vi "Lockin.vi"(4 "stop?":bool, 6 "initialize?":bool, 8 "error in (no error)":errorcluster, 11 "Transport":refnum<class "SMO.Transport.lvclass">) -> (0 "error out":errorcluster, 3 "Transport out":refnum<class "SMO.Transport.lvclass">)   [LabVIEW 2019, in "SMO.Transport.lvclass"]
uses:
  SMO.Transport.lvclass
  <userlib>/LevyLab/Instrument Framework/Instrument Types/Cryostat/Instrument.Cryostat.lvclass
  Control Experiment/Control Experiment.lvclass
  <userlib>/LevyLab/Krohn Hite 7008/Instrument.KH7008.lvclass
  <userlib>/LevyLab/Lockin-Multichannel/Instrument.Lockin/Instrument.Lockin.lvclass
  Control Experiment/Typedefs/Instruments--cluster.ctl
  <userlib>/LevyLab/Instrument Framework/Instrument Types/VSource/Instrument.VSource.lvclass
  <userlib>/LevyLab/Instrument Framework/Instrument Types/VNA/Instrument.VNA.lvclass
  <userlib>/LevyLab/Instrument Framework/Instrument Types/Strain/Instrument.Strain.lvclass
  <userlib>/LevyLab/Instrument Framework/Instrument Types/CBridge/Instrument.CBridge.lvclass
  SMO.SweepControl/SMO.SweepControl.lvclass
  SMO.Control Experiment/SMO.Control Experiment.lvclass
  C:/Program Files (x86)/National Instruments/LabVIEW 2019/user.lib/LevyLab/Instrument Framework/SMOs/Instrument/Instrument.lvclass
  C:/Program Files (x86)/National Instruments/LabVIEW 2019/vi.lib/JKI/JKI SMO/SMO/SMO.lvclass
  <userlib>/LevyLab/Instrument Framework/Instrument Types/Delay Line/Instrument.DelayLine.lvclass
panel:
  in  "Tab Control":enum32{"lockin/SG Control", "Data", "Other"}(tab)
  out "elapsed time (s)":u32=76
  in  "Experiment Comments":string="describe only the experiment you're doing right now"
  in  "Experiment Folder":string="Experiment folder"
  out "T (mK)":dbl
  out "Field (T)":dbl=0.5 format="%#_13g"
  out "time b/w points (ms)":u32=76
  in  "stop":bool
  out "x-y":u32
  out "X Lockins":cluster{dbl[], dbl[]}[](graph)
  out "Y Lockins":cluster{dbl[], dbl[]}[](graph)
  out "G4T":cluster{dbl[], dbl[]}[](graph)
  # "*** These controls are only read if this VI is the top level. If is is called from Sweep Control then the folder and comments come from Sweep Control.vi ***"
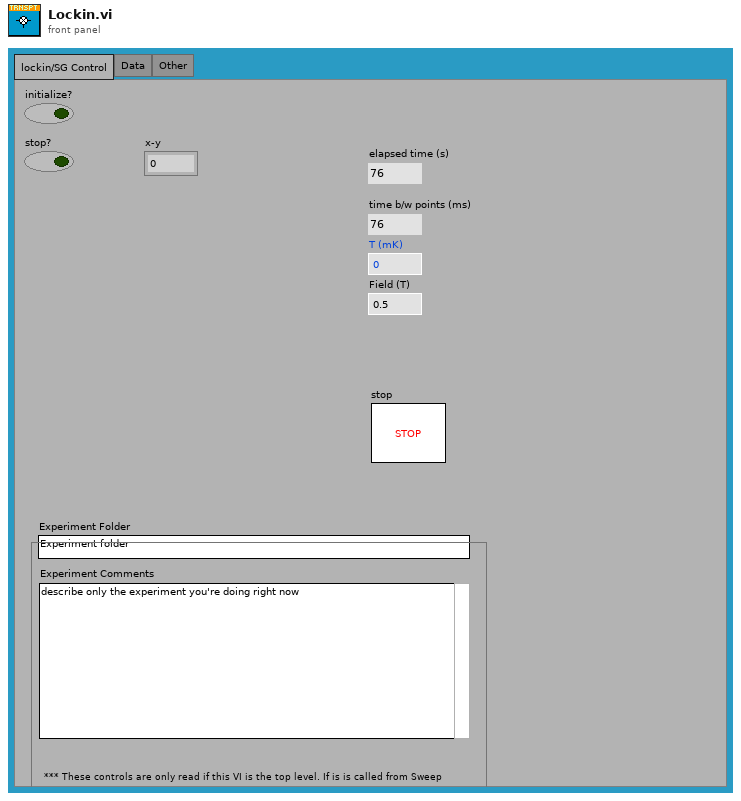
[diagram p1: front panel]
types:
  T1 = enum32{"Invalid", "Standard", "Closed", "Hidden", "Minimized", "Maximized"}
  T2 = enum32{"invalid app kind", "Development System", "Run Time System", "Student Edition", "Embedded LabVIEW", "Evaluation", "Custom"}
  T3 = typedef "Control Experiment.lvclass/Instruments--cluster.ctl" = cluster{"KH7008":refnum<class "Instrument.KH7008.lvclass">[], "Lockin":refnum<class "Instrument.Lockin.lvclass">, "Temperature":refnum<class "Instrument.Cryostat.lvclass">, "Magnet":refnum<class "Instrument.Cryostat.lvclass">, "Rotator":refnum<class "Instrument.Cryostat.lvclass">, "Level":refnum<class "Instrument.Cryostat.lvclass">, "Capacitance Bridge":refnum<class "Instrument.CBridge.lvclass">, "Delay Line":refnum<class "Instrument.DelayLine.lvclass">, "Strain Cell":refnum<class "Instrument.Strain.lvclass">, "VNA":refnum<class "Instrument.VNA.lvclass">, "Voltage Source":refnum<class "Instrument.VSource.lvclass">}
  T4 = cluster{"Core":cluster{"Current VI Reference":refnum<vi>, "Close Panel on Exit?":bool}, "Transport":refnum<class "SMO.Transport.lvclass">, "Control Experiment":refnum<class "SMO.Control Experiment.lvclass">, "Instruments":T3, "Results (Dictionary)":cluster{"key":string, "value":dbl}[], "ms [0]":u32, "ms [i]":u32, "Execution:State":enum32{"Bad", "Idle", "Run top level", "Running"}}
  T5 = enum32{"Bad", "Idle", "Run top level", "Running"}
  T6 = cluster{"Current VI Reference":refnum<vi>, "Close Panel on Exit?":bool}
  T7 = cluster{"I-":i32, "I+":i32, "V1-":i32, "V1+":i32, "I2-":i32, "I2+":i32, "V2-":i32, "V2+":i32}
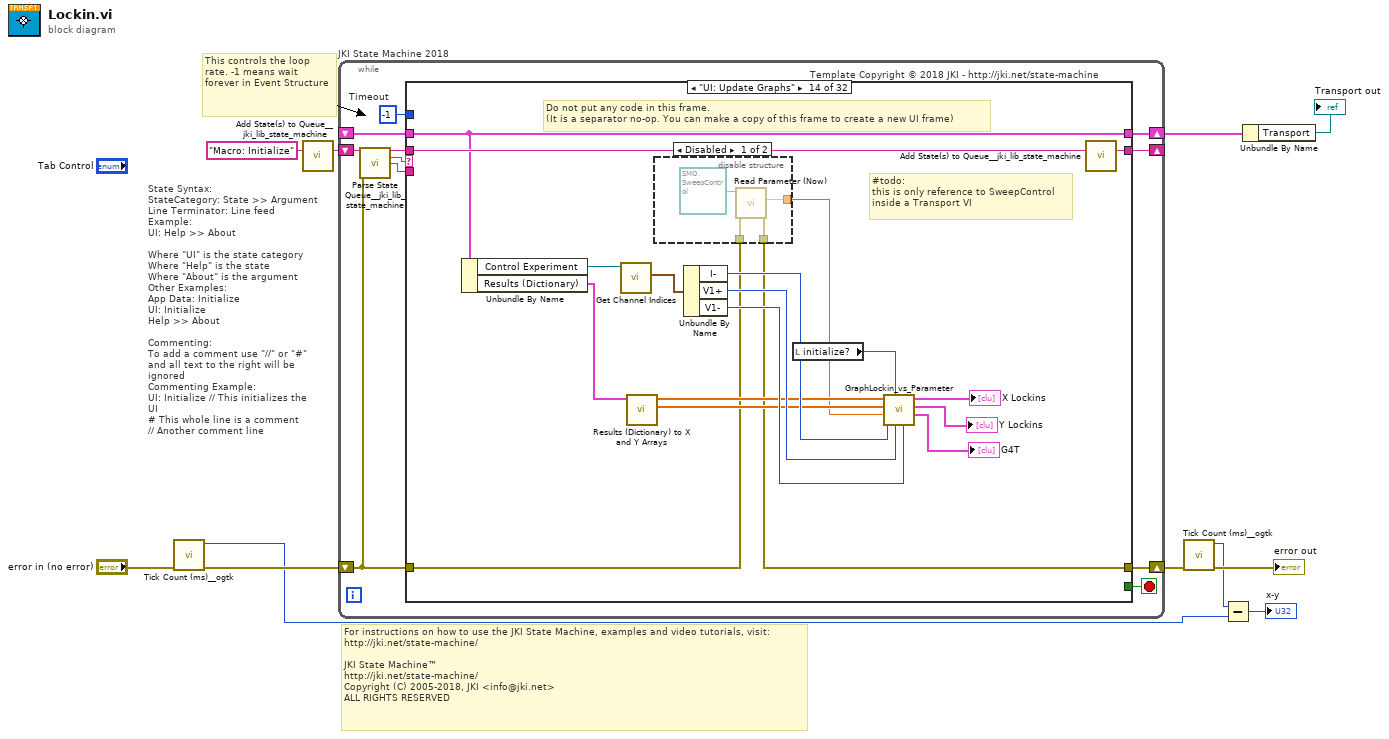
[diagram p0: block diagram]
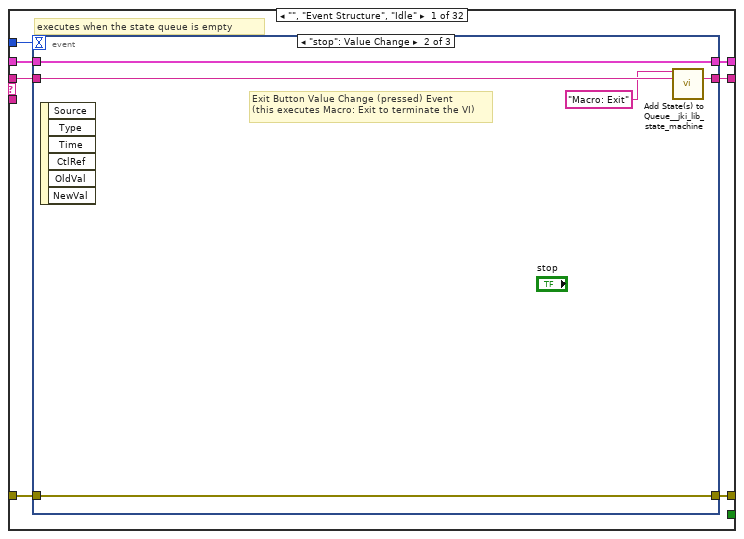
[diagram p2: hidden frame]
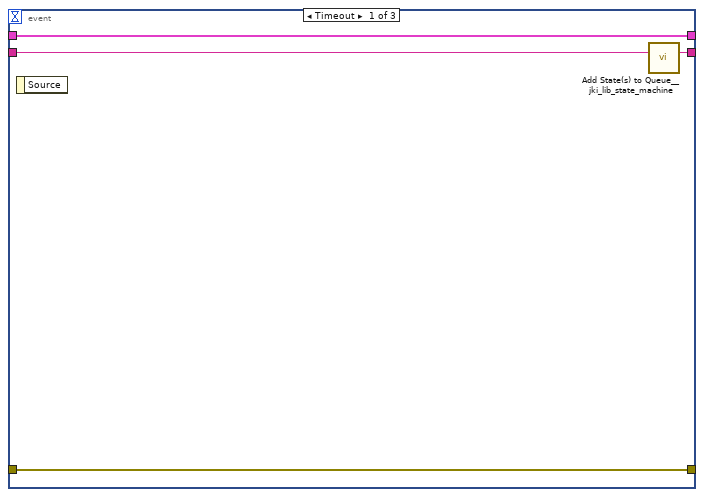
[diagram p3: hidden frame]
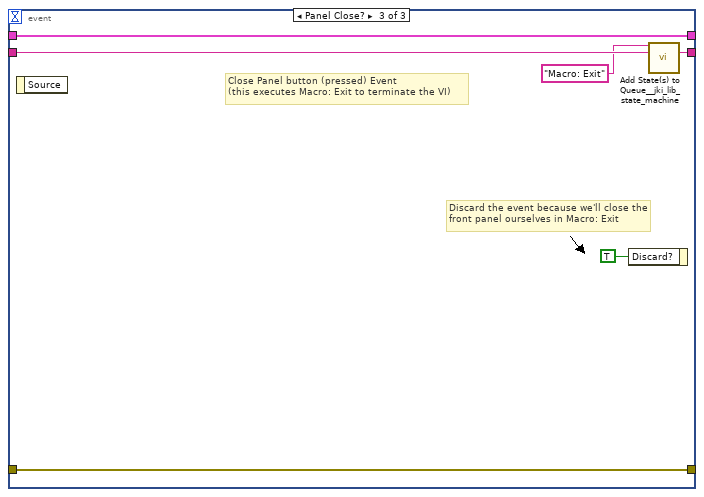
[diagram p4: hidden frame]
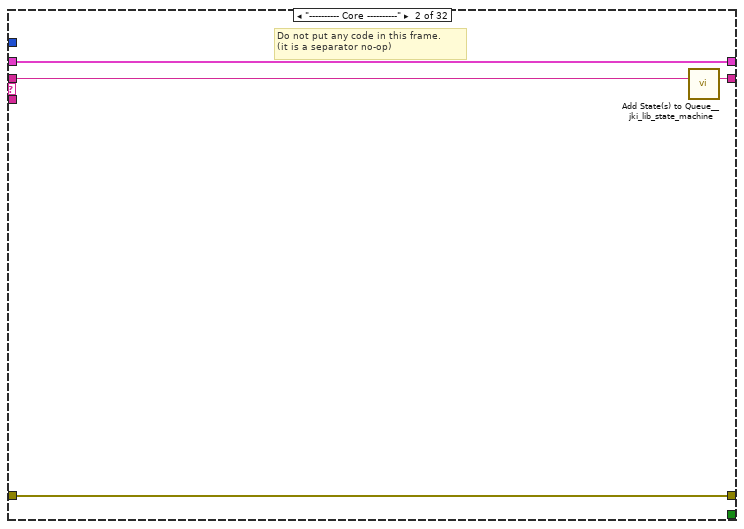
[diagram p5: hidden frame]
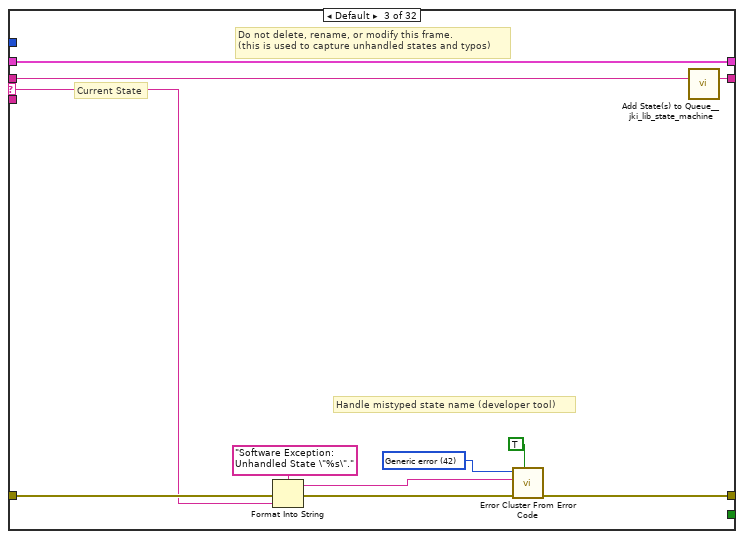
[diagram p6: hidden frame]
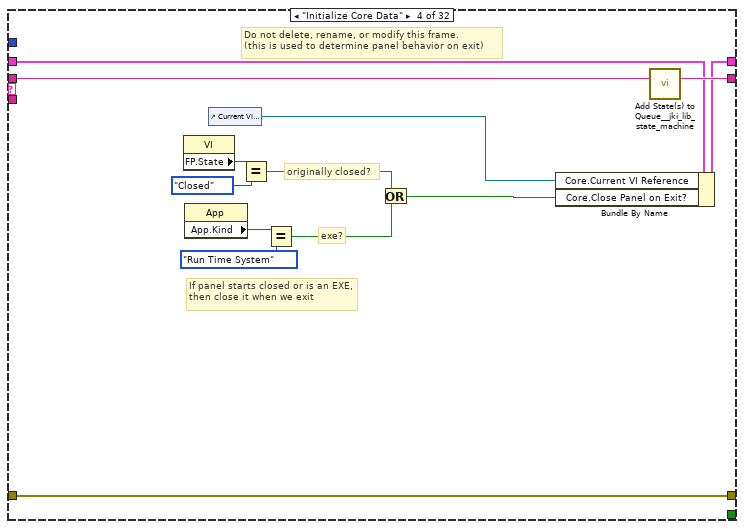
[diagram p7: hidden frame]
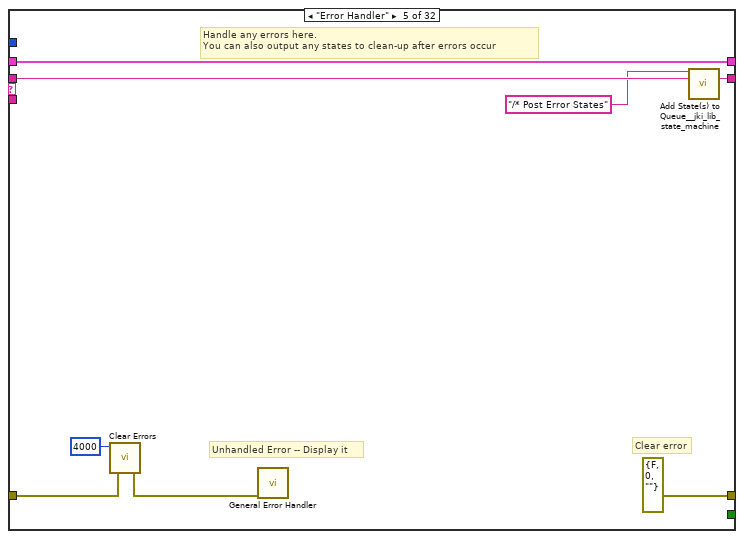
[diagram p8: hidden frame]
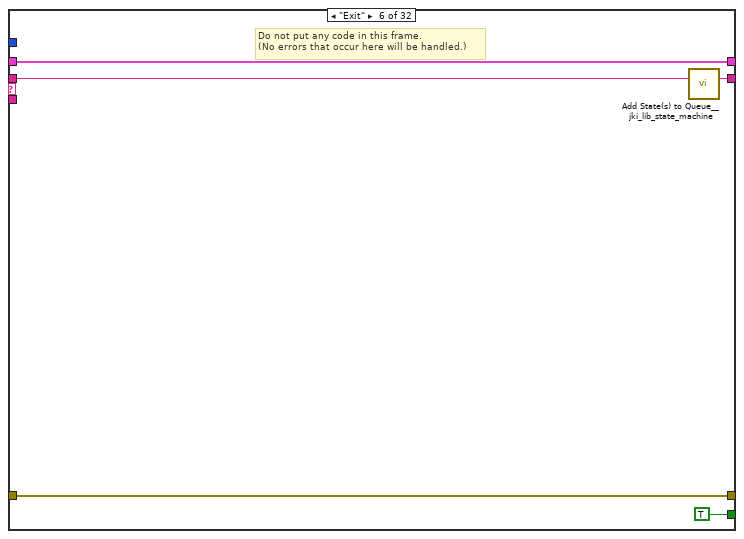
[diagram p9: hidden frame]
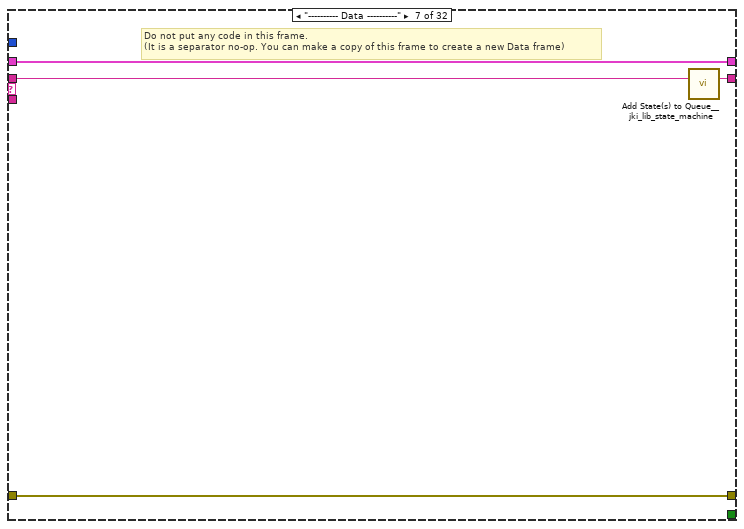
[diagram p10: hidden frame]
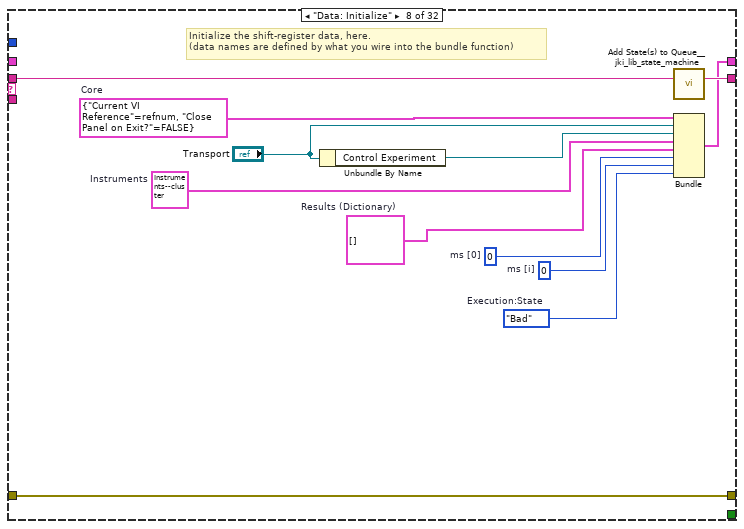
[diagram p11: hidden frame]
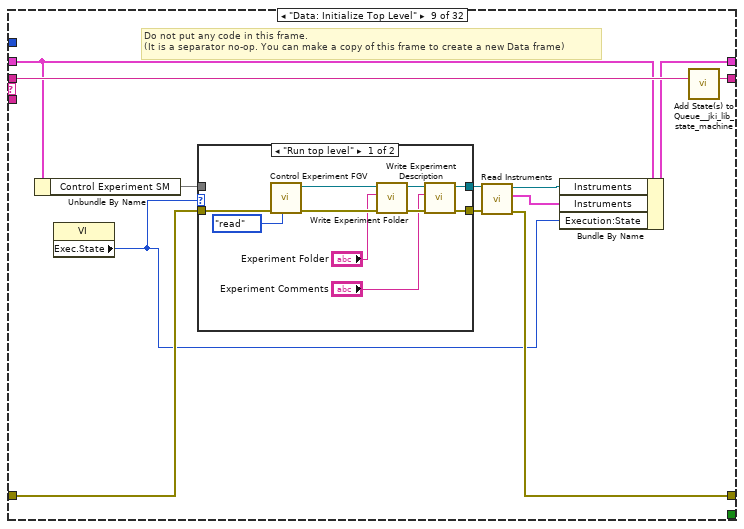
[diagram p12: hidden frame]
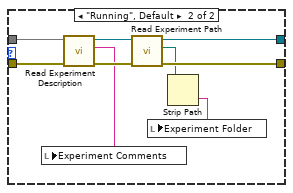
[diagram p13: hidden frame]
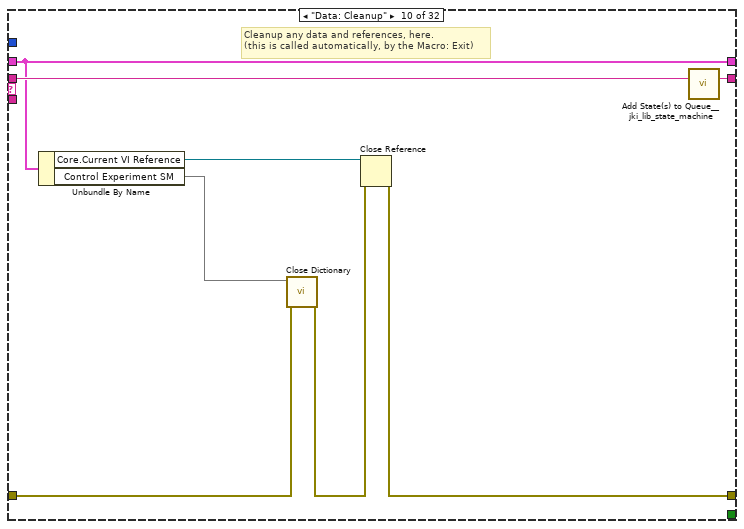
[diagram p14: hidden frame]
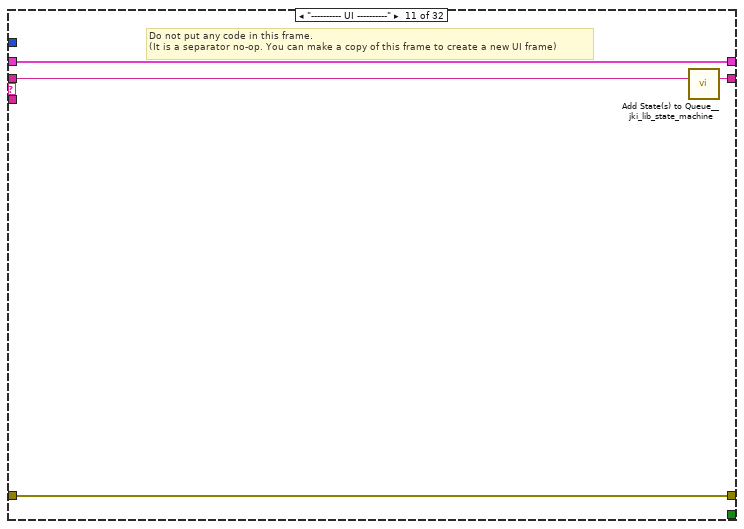
[diagram p15: hidden frame]
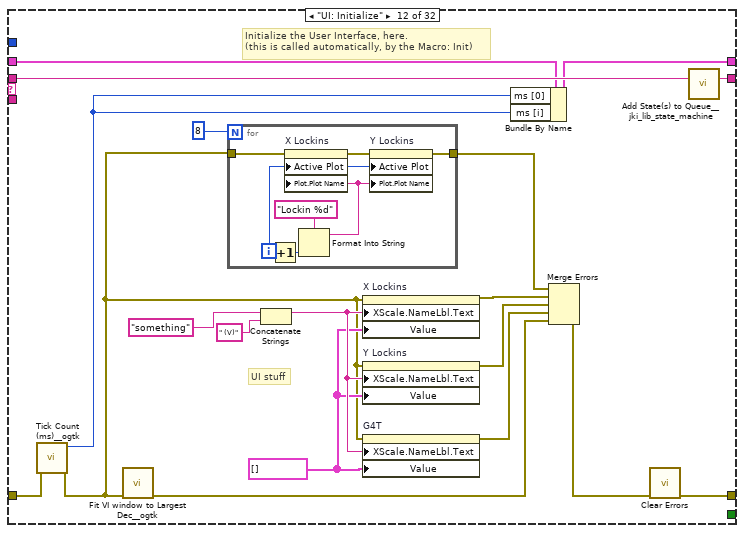
[diagram p16: hidden frame]
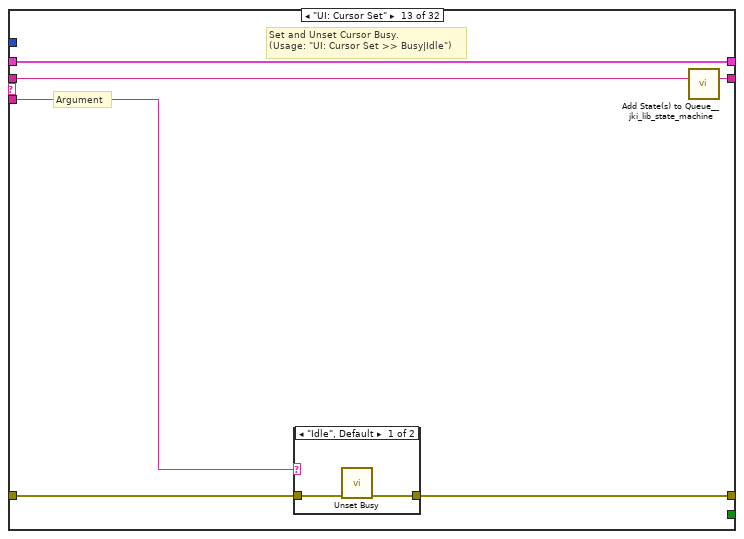
[diagram p17: hidden frame]
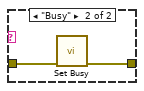
[diagram p18: hidden frame]
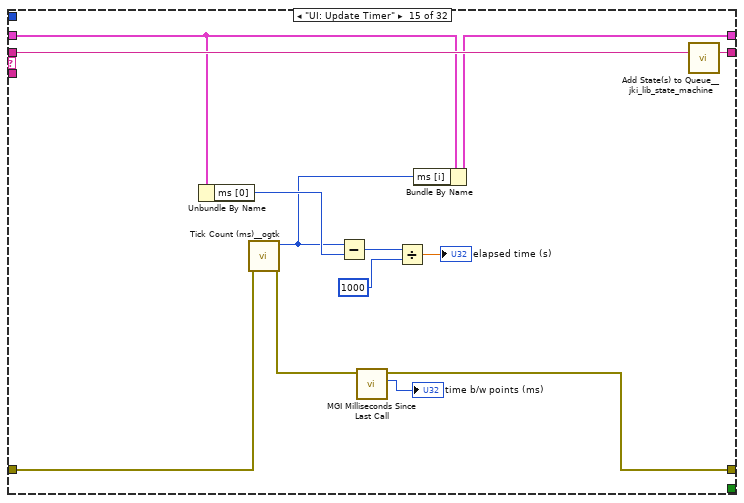
[diagram p20: hidden frame]
diagram:
  # "For instructions on how to use the JKI State Machine, examples and video tutorials, visit:\nhttp://jki.net/state-machine/\n\nJKI State Machine™\nhttp://jki.net/state-machine/\nCopyright (C) 2005-2018, JKI <info@jki.net>\nALL RIGHTS RESERVED"
  # "State Syntax:\nStateCategory: State >> Argument\nLine Terminator: Line feed\nExample:\nUI: Help >> About\n\nWhere \"UI\" is the state category\nWhere \"Help\" is the state\nWhere \"About\" is the argument\nOther Examples:\nApp Data: Initialize\nUI: Initialize\nHelp >> About\n\nCommenting:\nTo add a comment use \"//\" or \"#\" and all text to the right will be ignored\nCommenting Example:\nUI: Initialize // This initializes the UI\n# This whole line is a comment\n// Another comment line"
  # "This controls the loop rate. -1 means wait forever in Event Structure"
  n1 = call <userlib>:"Tick Count (ms)__ogtk.vi"("error in (no error)"="error in (no error)") -> ("error out"=w6:errorcluster, "millisecond timer value"=w2:u32)  [unwired: 9 in]
  n2 = call <vilib>:"Add State(s) to Queue__jki_lib_state_machine.vi"("State(s) in (\"\")"="Macro: Initialize") -> ("States Out"=w11:string)  [unwired: 14 in]
  n3 = while "JKI State Machine 2018" {
    shift-right: [w15] -> w9
    shift-left: _ -> [w14]
    shift-right: [w18] -> w5
    shift-left: w6 -> [w12]
    shift-right: [w17] -> _
    shift-left: w11 -> [w19]
    stop <- w16 stop-if-true
    w13 = -1  # Timeout
    # "Template Copyright © 2018 JKI - http://jki.net/state-machine"
    n4 = call <vilib>:"Parse State Queue__jki_lib_state_machine.vi"("State Queue"=w19, "Error In (no error)"=w12) -> ("Remaining States"=w21:string, "Current State"=w22:string, "Arguments"=w20:string)  [unwired: 11 in]
    n5 = case shown="\"UI: Update Graphs\"" w22 {
      selector: w22 -> [_ _ w49 _ _ _ _ _ _ _ _ _ _ _ _ _ _ _ _ _ _ _ _ _ _ _ _ _ _ _ _ _]
      tunnel: w21 -> [w29 w48 w53 w72 w80 w85 w89 w101 w113 w140 w144 w163 w176 w198 w216 w223 w292 w300 w314 w324 w328 w332 w338 w342 w354 w366 w378 w391 w418 w422 w426 w434]
      tunnel: w20 -> [_ _ _ _ _ _ _ _ _ _ _ _ w171 _ _ w217 _ _ _ _ _ _ _ _ _ _ _ _ _ _ _ _]
      tunnel: w14 -> [w27 w45 w51 w65 w77 w83 w86 _ w104 w136 w141 w150 w174 w186 w211 w219 w289 w298 w311 w321 w325 w329 w336 w339 w350 w363 w367 w386 w414 w419 w423 w432]
      tunnel: [w26 w46 w55 w69 errorcluster {"status"=FALSE, "code"=0, "source"=""} ("error out") w82 w87 w98 w105 w137 w142 w154 w172 w183 w205 w220 w290 w297 w312 w322 w326 w330 w334 w340 w346 w355 w369 w381 w409 w420 w424 w429] -> w18
      tunnel: w12 -> [w25 w46 w54 w69 w74 w82 w87 w98 w106 w134 w142 w151 w173 w184 w213 w221 w290 w297 w312 w322 w326 w330 w335 w340 w351 w360 w370 w389 w410 w420 w424 w430]
      tunnel: [w28 w47 w52 w71 w79 w84 w88 w100 w112 w139 w143 w162 w175 w197 w215 w222 w291 w299 w313 w323 w327 w331 w337 w341 w353 w365 w377 w390 w417 w421 w425 w433] -> w17
      tunnel: [_ _ _ _ _ TRUE _ _ _ _ _ _ _ _ _ _ _ _ _ _ _ _ _ _ _ _ _ _ _ _ _ _] -> w16
      tunnel: [w24 w45 w51 w70 w77 w83 w86 w99 w103 w136 w141 w149 w174 w186 w210 w219 w289 w298 w311 w321 w325 w329 w336 w339 w349 w362 w372 w387 w415 w419 w423 w432] -> w15
      tunnel: w13 -> [w23 _ _ _ _ _ _ _ _ _ _ _ _ _ _ _ _ _ _ _ _ _ _ _ _ _ _ _ _ _ _ _]
      frame "", "Event Structure", "Idle" {
        # "executes when the state queue is empty"
        n6 = event shown="[1] \"stop\": Value Change" {
          selector: _ -> [_ _ _]
          dyn-events: _ -> [_ _ _]
          timeout: w23 -> [_ _ _]
          tunnel: w29 -> [w33 w38 w44]
          tunnel: [w32 w37 w43] -> w28
          tunnel: w27 -> [w30 w35 w41]
          tunnel: [w31 w36 w42] -> w26
          tunnel: w25 -> [w31 w36 w42]
          tunnel: [w30 w35 w41] -> w24
          event Timeout {
            n7 = event-data() -> ()  [unwired: 1 in, 1 out]
            n8 = call <vilib>:"Add State(s) to Queue__jki_lib_state_machine.vi"("State(s) in (\"\")"=w33) -> ("States Out"=w32:string)  [unwired: 14 in]
          }
          event "stop": Value Change {
            # "Exit Button Value Change (pressed) Event\n(this executes Macro: Exit to terminate the VI)"
            n9 = event-data() -> ()  [unwired: 1 in, 6 out]
            n10 = call <vilib>:"Add State(s) to Queue__jki_lib_state_machine.vi"("State(s) in Front (\"\")"="Macro: Exit", "State(s) in (\"\")"=w38) -> ("States Out"=w37:string)  [unwired: 13 in]
          }
          event Panel Close? {
            # "Discard the event because we'll close the front panel ourselves in Macro: Exit"
            # "Close Panel button (pressed) Event\n(this executes Macro: Exit to terminate the VI)"
            n11 = event-data() -> ()  [unwired: 1 in, 1 out]
            n12 = event-data("Discard?"=TRUE) -> ()  [unwired: 1 in, 1 out]
            n13 = call <vilib>:"Add State(s) to Queue__jki_lib_state_machine.vi"("State(s) in Front (\"\")"="Macro: Exit", "State(s) in (\"\")"=w44) -> ("States Out"=w43:string)  [unwired: 13 in]
          }
        }
      }
      frame "---------- Core ----------" {
        # "Do not put any code in this frame.\n(it is a separator no-op)"
        n14 = call <vilib>:"Add State(s) to Queue__jki_lib_state_machine.vi"("State(s) in (\"\")"=w48) -> ("States Out"=w47:string)  [unwired: 14 in]
      }
      frame Default {
        w58 = 42 items=["No error", "Argument error", "Memory is full", "Out of zone", "End of file", "File already open", "Generic file I/O error", "File not found", "File permission error", "Disk is full", "Duplicate path", "Too many files open", "System feature not enabled", "Resource file not found", "Cannot add resource", "Resource not found", "Image not found", "Image memory error", "Pen does not exist", "Config type invalid", "Config token not found", "Config parse error", "Config memory error", "Bad external code format", "Bad external code offset", "External code not present", "Null window", "Destroy window error", "Null menu", "Print aborted", "Bad print record", "Print driver error", "Windows error during printing", "Memory error during printing", "Print dialog error", "Generic print error", "Invalid device refnum", "Device not found", "Device parameter error", "Device unit error", "Cannot open device", "Device call aborted", "Generic error", "Cancelled by user", "Object ID too low", "Object ID too high", "Object not in heap", "Unknown heap", "Unknown object (invalid DefProc)", "Unknown object (DefProc not in table)", "Message out of range", "Invalid (null) method", "Unknown message", "Manager call not supported", "Bad address", "Network operation in progress", "Network operation timed out", "Connection is busy", "Network attribute not supported", "Network error", "Address in use", "System out of memory", "Connection aborted", "Connection refused", "Not connected", "Already connected", "Connection closed", "Initialization error (interapplication manager)", "Bad occurrence", "Wait on unbound occurrence handler", "Occurrence queue overflow", "Datalog type conflict", "Unused", "Unrecognized type (interapplication manager)", "Memory corrupt", "Failed to make temporary DLL", "Old CIN version", "Drag socket not found", "Failed to load drop-object", "Failed to register OLE object", "Failed to release OLE object", "Format specifier type mismatch", "Unknown format specifier", "Too few format specifiers", "Too many format specifiers", "Scan failed", "Newer CIN version", "Error converting to variant", "Runtime menu error", "Password tampered", "Variant attribute not found", "Incompatible variant data type", "Event data is not available", "Event Store is not present", "Occurrence is not found", "Event Queue is not created", "Event info is not available", "Refnum passed is NULL", "Error retrieving Class GUID", "Error retrieving CoClass GUID", "Error retrieving TypeLib GUID.", "Bad built application magic bytes.", "Specific driver is different from the specific driver associated with the Logical Name.", "There is no session opened to the class driver.", "Max Error", "MAX - Error with config objects", "MAX - Error loading configuration", "MAX - Group not supported"]
        # "Current State"
        # "Do not delete, rename, or modify this frame.\n(this is used to capture unhandled states and typos)"
        # "Handle mistyped state name (developer tool)"
        n15 = Format Into String(format string="Software Exception: Unhandled State \"%s\"." ("message"), error in=w54, w49) -> (resulting string=w57:string, error out=w56:errorcluster)  [unwired: 1 in]
        n16 = call <vilib>:"Error Cluster From Error Code.vi"("show call chain? (False)"=TRUE, "error in (no error)"=w56, "error message (\"\")"=w57, "error code (0)"=w58) -> ("error out"=w55:errorcluster)  [unwired: 5 in]
        n17 = call <vilib>:"Add State(s) to Queue__jki_lib_state_machine.vi"("State(s) in (\"\")"=w53) -> ("States Out"=w52:string)  [unwired: 14 in]
      }
      frame "Initialize Core Data" {
        # "Do not delete, rename, or modify this frame.\n(this is used to determine panel behavior on exit)"
        # "originally closed?"
        # "exe?"
        # "If panel starts closed or is an EXE, then close it when we exit"
        n18 = property class="VI"() -> ("FP.State"=w62:T1)  [unwired: 2 in, 2 out]
        n19 = property class="App"() -> ("App.Kind"=w68:T2)  [unwired: 2 in, 2 out]
        n20 = control-ref of="Current VI Reference"() -> (w63:refnum<vi>)
        n21 = Equal?(x=w62, y=T1."Closed" ("Front Panel Window:State")) -> (x = y?=w60:bool)
        n22 = Equal?(x=w68, y=T2."Run Time System" ("Application:Kind")) -> (x = y?=w66:bool)
        n23 = Or(x=w60, y=w66) -> (x .or. y?=w64:bool)
        n24 = Bundle By Name(cluster=w65, "Core.Current VI Reference"=w63, "Core.Close Panel on Exit?"=w64) -> (w70:T4)
        n25 = call <vilib>:"Add State(s) to Queue__jki_lib_state_machine.vi"("State(s) in (\"\")"=w72) -> ("States Out"=w71:string)  [unwired: 14 in]
      }
      frame "Error Handler" {
        # "Unhandled Error -- Display it"
        # "Handle any errors here.\nYou can also output any states to clean-up after errors occur"
        # "Clear error"
        n26 = call <vilib>:"Clear Errors.vi"("error in (no error)"=w74, "specific error code to clear (0: all)"=4000) -> ("error out"=w73:errorcluster)  [unwired: 4 in, 1 out]
        n27 = call <vilib>:"General Error Handler.vi"("error in (no error)"=w73) -> ()  [unwired: 10 in, 5 out]
        n28 = call <vilib>:"Add State(s) to Queue__jki_lib_state_machine.vi"("State(s) in Front (\"\")"="/* Post Error States", "State(s) in (\"\")"=w80) -> ("States Out"=w79:string)  [unwired: 13 in]
      }
      frame "Exit" {
        # "Do not put any code in this frame.\n(No errors that occur here will be handled.)"
        n29 = call <vilib>:"Add State(s) to Queue__jki_lib_state_machine.vi"("State(s) in (\"\")"=w85) -> ("States Out"=w84:string)  [unwired: 14 in]
      }
      frame "---------- Data ----------" {
        # "Do not put any code in this frame.\n(It is a separator no-op. You can make a copy of this frame to create a new Data frame)"
        n30 = call <vilib>:"Add State(s) to Queue__jki_lib_state_machine.vi"("State(s) in (\"\")"=w89) -> ("States Out"=w88:string)  [unwired: 14 in]
      }
      frame "Data: Initialize" {
        w90 = cluster{"key":string, "value":dbl}[] []  # Results (Dictionary)
        w91 = T5."Bad"  # Execution:State
        w93 = u32 0  # ms [i]
        w94 = u32 0  # ms [0]
        w95 = T3 {"KH7008"=[], "Lockin"=refnum, "Temperature"=refnum, "Magnet"=refnum, "Rotator"=refnum, "Level"=refnum, "Capacitance Bridge"=refnum, "Delay Line"=refnum, "Strain Cell"=refnum, "VNA"=refnum, "Voltage Source"=refnum}  # Instruments
        w97 = T6 {"Current VI Reference"=refnum, "Close Panel on Exit?"=FALSE}  # Core
        # "Initialize the shift-register data, here.\n(data names are defined by what you wire into the bundle function)"
        n31 = Unbundle By Name("Transport") -> ("Control Experiment"=w92:refnum<class "SMO.Control Experiment.lvclass">)
        n32 = call <vilib>:"Add State(s) to Queue__jki_lib_state_machine.vi"("State(s) in (\"\")"=w101) -> ("States Out"=w100:string)  [unwired: 14 in]
        n33 = Bundle("Core"=w97, "Transport"="Transport", "Control Experiment"=w92, "Instruments"=w95, "Results (Dictionary)"=w90, "ms [0]"=w94, "ms [i]"=w93, "Execution:State"=w91) -> (w99:T4)  [unwired: 1 in]
      }
      frame "Data: Initialize Top Level" {
        # "Do not put any code in this frame.\n(It is a separator no-op. You can make a copy of this frame to create a new Data frame)"
        n34 = Unbundle By Name(w104) -> ("Control Experiment SM"=w107)
        n35 = property class="VI"() -> ("Exec.State"=w102:T5)  [unwired: 2 in, 2 out]
        n36 = case shown="\"Run top level\"" w102 {
          tunnel: w106 -> [w123 w131]
          tunnel: [w118 w127] -> w108
          tunnel: [w117 w128] -> w109
          tunnel: w107 -> [_ w132]
          frame "Run top level" {
            n37 = call "Control Experiment FGV.vi"("Function"=enum16{"read", "write"}."read", "error in (no error)"=w123) -> ("error out"=w121:errorcluster, "Control Experiment.lvclass out"=w122:refnum<class "Control Experiment.lvclass">)  [unwired: 8 in]
            n38 = call "Write Experiment Folder.vi"("error in (no error)"=w121, "Experiment Folder"="Experiment Folder", "Control Experiment in"=w122) -> ("error out"=w119:errorcluster, "Control Experiment out"=w120:refnum<class "Control Experiment.lvclass">)  [unwired: 7 in]
            n39 = call "Write Experiment Description.vi"("error in (no error)"=w119, "Experiment Description"="Experiment Comments", "Control Experiment in"=w120) -> ("error out"=w118:errorcluster, "Control Experiment out"=w117:refnum<class "Control Experiment.lvclass">)  [unwired: 7 in]
          }
          frame "Running", Default {
            n40 = call "Read Experiment Description.vi"("error in (no error)"=w131, "Control Experiment in"=w132) -> ("error out"=w130:errorcluster, "Experiment Description"=w125:string, "Control Experiment out"=w129:refnum<class "Control Experiment.lvclass">)  [unwired: 7 in]
            n41 = local write "Experiment Comments"(w125) -> ()
            n42 = call "Read Experiment Path.vi"("error in (no error)"=w130, "Control Experiment in"=w129) -> ("error out"=w127:errorcluster, "Experiment Path"=w126:path, "Control Experiment out"=w128:refnum<class "Control Experiment.lvclass">)  [unwired: 7 in]
            n43 = Strip Path(path=w126) -> (name=w124:string)  [unwired: 1 out]
            n44 = local write "Experiment Folder"(w124) -> ()
          }
        }
        n45 = call "Read Instruments.vi"("error in (no error)"=w108, "Control Experiment in"=w109) -> ("error out"=w105:errorcluster, "Instruments"=w111:T3, "Control Experiment out"=w110:refnum<class "Control Experiment.lvclass">)  [unwired: 7 in]
        n46 = Bundle By Name(cluster=w104, "Instruments"=w110, "Instruments"=w111, "Execution:State"=w102) -> (w103:T4)
        n47 = call <vilib>:"Add State(s) to Queue__jki_lib_state_machine.vi"("State(s) in (\"\")"=w113) -> ("States Out"=w112:string)  [unwired: 14 in]
      }
      frame "Data: Cleanup" {
        # "Cleanup any data and references, here.\n(this is called automatically, by the Macro: Exit)"
        n48 = Unbundle By Name(w136) -> ("Core.Current VI Reference"=w138:refnum<vi>, "Control Experiment SM"=w135)
        n49 = call "Close Dictionary.vi"("error in (no error)"=w134, "Control Experiment in"=w135) -> ("error out"=w133:errorcluster)  [unwired: 8 in, 1 out]
        n50 = Close Reference(reference=w138, error in (no error)=w133) -> (error out=w137:errorcluster)
        n51 = call <vilib>:"Add State(s) to Queue__jki_lib_state_machine.vi"("State(s) in (\"\")"=w140) -> ("States Out"=w139:string)  [unwired: 14 in]
      }
      frame "---------- UI ----------" {
        # "Do not put any code in this frame.\n(It is a separator no-op. You can make a copy of this frame to create a new UI frame)"
        n52 = call <vilib>:"Add State(s) to Queue__jki_lib_state_machine.vi"("State(s) in (\"\")"=w144) -> ("States Out"=w143:string)  [unwired: 14 in]
      }
      frame "UI: Initialize" {
        w147 = cluster{dbl[], dbl[]}[] [] ("G4T")
        # "UI stuff"
        # "Initialize the User Interface, here.\n(this is called automatically, by the Macro: Init)"
        n53 = call <userlib>:"Tick Count (ms)__ogtk.vi"("error in (no error)"=w151) -> ("error out"=w145:errorcluster, "millisecond timer value"=w148:u32)  [unwired: 9 in]
        n54 = call <userlib>:"Fit VI window to Largest Dec__ogtk.vi"("error in (no error)"=w145) -> ("error out"=w153:errorcluster)  [unwired: 5 in, 1 out]
        n55 = for {
          N: 8 -> [_]
          tunnel: [w164] -> w158
          tunnel: w145 -> [w169]
          i -> [w167]
          n56 = Increment(x=w167) -> (x+1=w165:i32)
          n57 = Format Into String(format string="Lockin %d", w165) -> (resulting string=w168:string)  [unwired: 2 in, 1 out]
          n58 = property on="X Lockins" class="XYGraph (strict)"(error in=w169, "Active Plot"=w167, "Plot.Plot Name"=w168) -> (error out=w166:errorcluster)  [unwired: 1 in, 1 out]
          n59 = property on="Y Lockins" class="XYGraph (strict)"(error in=w166, "Active Plot"=w167, "Plot.Plot Name"=w168) -> (error out=w164:errorcluster)  [unwired: 1 in, 1 out]
        }
        n60 = Concatenate Strings("something" ("string"), " (V)" ("string")) -> (w157:string)
        n61 = property on="X Lockins" class="XYGraph (strict)"(error in=w145, "XScale.NameLbl.Text"=w157, "Value"=w147) -> (error out=w159:errorcluster)  [unwired: 1 in, 1 out]
        n62 = property on="Y Lockins" class="XYGraph (strict)"(error in=w145, "XScale.NameLbl.Text"=w157, "Value"=w147) -> (error out=w160:errorcluster)  [unwired: 1 in, 1 out]
        n63 = property on="G4T" class="XYGraph (strict)"(error in=w145, "XScale.NameLbl.Text"=w157, "Value"=w147) -> (error out=w161:errorcluster)  [unwired: 1 in, 1 out]
        n64 = Bundle By Name(cluster=w150, "ms [0]"=w148, "ms [i]"=w148) -> (w149:T4)
        n65 = Merge Errors(w158, w159, w160, w161, w153) -> (w152:errorcluster)
        n66 = call <vilib>:"Clear Errors.vi"("error in (no error)"=w152) -> ("error out"=w154:errorcluster)  [unwired: 5 in, 1 out]
        n67 = call <vilib>:"Add State(s) to Queue__jki_lib_state_machine.vi"("State(s) in (\"\")"=w163) -> ("States Out"=w162:string)  [unwired: 14 in]
      }
      frame "UI: Cursor Set" {
        # "Argument"
        # "Set and Unset Cursor Busy.\n(Usage: \"UI: Cursor Set >> Busy|Idle\")"
        n68 = case shown="\"Idle\", Default" w171 {
          tunnel: w173 -> [w178 w180]
          tunnel: [w177 w179] -> w172
          frame "Idle", Default {
            n69 = call <vilib>:"Unset Busy.vi"("error in (no error)"=w178) -> ("error out"=w177:errorcluster)  [unwired: 10 in]
          }
          frame "Busy" {
            n70 = call <vilib>:"Set Busy.vi"("error in (no error)"=w180) -> ("error out"=w179:errorcluster)  [unwired: 9 in, 1 out]
          }
        }
        n71 = call <vilib>:"Add State(s) to Queue__jki_lib_state_machine.vi"("State(s) in (\"\")"=w176) -> ("States Out"=w175:string)  [unwired: 14 in]
      }
      frame "UI: Update Graphs" {
        # "#todo:\nthis is only reference to SweepControl\ninside a Transport VI"
        # "Do not put any code in this frame.\n(It is a separator no-op. You can make a copy of this frame to create a new UI frame)"
        n72 = Unbundle By Name(w186) -> ("Control Experiment"=w195:refnum<class "SMO.Control Experiment.lvclass">, "Results (Dictionary)"=w181:cluster{"key":string, "value":dbl}[])
        n73 = call "Get Channel Indices.vi"("Control Experiment in"=w195) -> ("Indices"=w194:T7)  [unwired: 8 in, 2 out]
        n74 = call "Results (Dictionary) to X and Y Arrays.vi"("Results (Dictionary)"=w181) -> ("Y"=w187:dbl[], "X"=w188:dbl[])  [unwired: 9 in]
        n75 = disable-structure shown="Disabled" {
          disable-tunnel: w184 -> [w202 w203]
          disable-tunnel: [w201 w203] -> w183
          disable-tunnel: [w200 _] -> w182
          frame Disabled {
            n76 = call "Read Parameter (Now).vi"("error in (no error)"=w202, "SweepControl in"=refnum<class "SMO.SweepControl.lvclass"> refnum) -> ("error out"=w201:errorcluster, "Parameter (Now)"=w200:dbl)  [unwired: 7 in, 1 out]
          }
          frame Enabled {
          }
        }
        n77 = Unbundle By Name(w194) -> ("I-"=w191:i32, "V1+"=w193:i32, "V1-"=w192:i32)
        n78 = local read "initialize?"() -> (w185:bool)
        n79 = call "GraphLockin_vs_Parameter.vi"("V-"=w192, "V+"=w193, "reset?"=w185, "Current"=w191, "Parameter"=w182, "Y[ ]"=w187, "X[ ]"=w188) -> ("G(e2/h) vs Parameter"=→"G4T":cluster{"Y":dbl[], "Y":dbl[]}[], "Y vs Parameter"=→"Y Lockins":cluster{dbl[], dbl[]}[], "X vs Parameter"=→"X Lockins":cluster{dbl[], dbl[]}[])  [unwired: 1 in, 1 out]
        n80 = call <vilib>:"Add State(s) to Queue__jki_lib_state_machine.vi"("State(s) in (\"\")"=w198) -> ("States Out"=w197:string)  [unwired: 14 in]
      }
      frame "UI: Update Timer" {
        n81 = Unbundle By Name(w211) -> ("ms [0]"=w212:u32)
        n82 = call <userlib>:"Tick Count (ms)__ogtk.vi"("error in (no error)"=w213) -> ("error out"=w206:errorcluster, "millisecond timer value"=w204:u32)  [unwired: 9 in]
        n83 = Subtract(x=w204, y=w212) -> (x-y=w208:u32)
        n84 = call <userlib>:"MGI Milliseconds Since Last Call.vi"("Error In"=w206) -> ("ms"=→"time b/w points (ms)":u32, "Error Out"=w205:errorcluster)  [unwired: 5 in]
        n85 = Divide(x=w208, y=u32 1000 ("x")) -> (x/y=→"elapsed time (s)":dbl)
        n86 = Bundle By Name(cluster=w211, "ms [i]"=w204) -> (w210:T4)
        n87 = call <vilib>:"Add State(s) to Queue__jki_lib_state_machine.vi"("State(s) in (\"\")"=w216) -> ("States Out"=w215:string)  [unwired: 14 in]
      }
      frame "UI: Front Panel State" {
        # "Argument"
        # "Set Front Panel Open or Closed\n(Usage: \"UI: Front Panel State >> Open|Close\")"
        n88 = Unbundle By Name(w219) -> ("Core.Current VI Reference"=w218:refnum<vi>)
        n89 = case shown="\"Minimize\", \"Minimized\"" w217 {
          tunnel: w221 -> [w229 w244 w255 w268 w281]
          tunnel: [w231 w245 w257 w270 w283] -> w220
          tunnel: w218 -> [w230 w242 w256 w269 w282]
          frame "Open", "Standard", Default {
            w224 = T1."Standard" ("State")
            n90 = property class="VI"(reference=w230, error in=w229) -> (reference out=w227:refnum<vi>, error out=w228:errorcluster, "FP.State"=w226:T1)
            n91 = Not Equal?(x=w226, y=w224) -> (x != y?=w225:bool)
            n92 = case shown="True" w225 {
              tunnel: [w235 w237] -> w231
              tunnel: w228 -> [w234 w237]
              tunnel: w227 -> [w233 _]
              tunnel: w224 -> [w232 _]
              frame True {
                n93 = invoke class="VI" method="FP.Open"(reference=w233, error in=w234, "Activate"=TRUE, "State"=w232) -> (error out=w235:errorcluster)  [unwired: 1 in, 4 out]
              }
              frame False {
              }
            }
          }
          frame "Close", "Closed" {
            n94 = property class="VI"(reference=w242, error in=w244) -> (reference out=w241:refnum<vi>, error out=w243:errorcluster, "FP.State"=w239:T1)
            n95 = Not Equal?(x=w239, y=T1."Closed" ("Front Panel Window:State")) -> (x != y?=w238:bool)
            n96 = case shown="True" w238 {
              tunnel: [w246 w249] -> w245
              tunnel: w243 -> [w246 w248]
              tunnel: w241 -> [_ w247]
              frame False {
              }
              frame True {
                n97 = invoke class="VI" method="FP.Close"(reference=w247, error in=w248) -> (error out=w249:errorcluster)  [unwired: 1 in, 2 out]
              }
            }
          }
          frame "Hidden", "Hide" {
            w250 = T1."Hidden" ("State")
            n98 = property class="VI"(reference=w256, error in=w255) -> (reference out=w253:refnum<vi>, error out=w254:errorcluster, "FP.State"=w252:T1)
            n99 = Not Equal?(x=w252, y=w250) -> (x != y?=w251:bool)
            n100 = case shown="True" w251 {
              tunnel: [w261 w262] -> w257
              tunnel: w254 -> [w260 w262]
              tunnel: w253 -> [w259 _]
              tunnel: w250 -> [w258 _]
              frame True {
                n101 = invoke class="VI" method="FP.Open"(reference=w259, error in=w260, "State"=w258) -> (error out=w261:errorcluster)  [unwired: 2 in, 4 out]
              }
              frame False {
              }
            }
          }
          frame "Minimize", "Minimized" {
            w263 = T1."Minimized" ("State")
            n102 = property class="VI"(reference=w269, error in=w268) -> (reference out=w266:refnum<vi>, error out=w267:errorcluster, "FP.State"=w265:T1)
            n103 = Not Equal?(x=w265, y=w263) -> (x != y?=w264:bool)
            n104 = case shown="True" w264 {
              tunnel: [w274 w275] -> w270
              tunnel: w267 -> [w273 w275]
              tunnel: w266 -> [w272 _]
              tunnel: w263 -> [w271 _]
              frame True {
                n105 = invoke class="VI" method="FP.Open"(reference=w272, error in=w273, "State"=w271) -> (error out=w274:errorcluster)  [unwired: 2 in, 4 out]
              }
              frame False {
              }
            }
          }
          frame "Maximize", "Maximized" {
            w276 = T1."Maximized" ("State")
            n106 = property class="VI"(reference=w282, error in=w281) -> (reference out=w279:refnum<vi>, error out=w280:errorcluster, "FP.State"=w278:T1)
            n107 = Not Equal?(x=w278, y=w276) -> (x != y?=w277:bool)
            n108 = case shown="True" w277 {
              tunnel: [w287 w288] -> w283
              tunnel: w280 -> [w286 w288]
              tunnel: w279 -> [w285 _]
              tunnel: w276 -> [w284 _]
              frame True {
                n109 = invoke class="VI" method="FP.Open"(reference=w285, error in=w286, "State"=w284) -> (error out=w287:errorcluster)  [unwired: 2 in, 4 out]
              }
              frame False {
              }
            }
          }
        }
        n110 = call <vilib>:"Add State(s) to Queue__jki_lib_state_machine.vi"("State(s) in (\"\")"=w223) -> ("States Out"=w222:string)  [unwired: 14 in]
      }
      frame "---------- Macro ----------" {
        # "Do not put any code in this frame.\n(It is a separator no-op. You can make a copy of this frame to create a new Macro frame)"
        n111 = call <vilib>:"Add State(s) to Queue__jki_lib_state_machine.vi"("State(s) in (\"\")"=w292) -> ("States Out"=w291:string)  [unwired: 14 in]
      }
      frame "Macro: Initialize" {
        # "Initialization Macro\n(This is called once, when the VI starts)"
        n112 = Select(t="Data: Initialize\nInitialize Core Data\nUI: Initialize\nUI: Front Panel State >> Open\nData: Initialize Top Level\nConfigure: Wait\nMeasure: Temperature\nMeasure: Magnet\nMeasure: Capacitance\nMacro: Sweep", s="initialize?", f="Data: Initialize\nInitialize Core Data\nMacro: Sweep") -> (s? t:f=w293:string)
        n113 = call <vilib>:"Add State(s) to Queue__jki_lib_state_machine.vi"("State(s) in Front (\"\")"=w293, "State(s) in (\"\")"=w300) -> ("States Out"=w299:string)  [unwired: 13 in]
      }
      frame "Macro: Sweep" {
        # "stop if true"
        n114 = local read "stop"() -> (w306:bool)
        n115 = Or(x=w306, y="stop?") -> (x .or. y?=w307:bool)
        n116 = Select(t="File: Save" ("State(s) in Front (\"\")"), s=w307, f="" ("State(s) in Front (\"\")")) -> (s? t:f=w302:string)
        n117 = call <vilib>:"Add State(s) to Queue__jki_lib_state_machine.vi"("State(s) in Front (\"\")"=w302, "State(s) at Back (\"\")"="Macro: Exit" ("State(s) in Front (\"\")")) -> ("States Out"=w301:string)  [unwired: 13 in]
        n118 = call <vilib>:"Add State(s) to Queue__jki_lib_state_machine.vi"("State(s) in Front (\"\")"="Measure: Lockin\nMeasure: Time\n//Measure: Temperature\nUI: Update Graphs\nUI: Update Timer" ("State(s) in Front (\"\")"), "State(s) at Back (\"\")"=w301) -> ("States Out"=w309:string)  [unwired: 13 in]
        n119 = call <vilib>:"Add State(s) to Queue__jki_lib_state_machine.vi"("State(s) in (\"\")"=w314, "State(s) at Back (\"\")"=w309) -> ("States Out"=w313:string)  [unwired: 13 in]
      }
      frame "Macro: Exit" {
        # "Exit Macro\n(This is called once, when the VI exits)"
        n120 = Unbundle By Name(w321) -> ("Core.Close Panel on Exit?"=w320:bool)
        n121 = Select(t="UI: Front Panel State >> Close", s=w320, f="") -> (s? t:f=w317:string)
        n122 = call <vilib>:"Add State(s) to Queue__jki_lib_state_machine.vi"("State(s) in (\"\")"=w317, "State(s) at Back (\"\")"="Data: Cleanup\nExit") -> ("States Out"=w315:string)  [unwired: 13 in]
        n123 = call <vilib>:"Add State(s) to Queue__jki_lib_state_machine.vi"("State(s) in Front (\"\")"=w315, "State(s) in (\"\")"=w324) -> ("States Out"=w323:string)  [unwired: 13 in]
      }
      frame "---------- Sweep ----------" {
        # "Do not put any code in this frame.\n(It is a separator no-op. You can make a copy of this frame to create a new Macro frame)"
        n124 = call <vilib>:"Add State(s) to Queue__jki_lib_state_machine.vi"("State(s) in (\"\")"=w328) -> ("States Out"=w327:string)  [unwired: 14 in]
      }
      frame "---------- Configure ----------" {
        # "Do not put any code in this frame.\n(It is a separator no-op. You can make a copy of this frame to create a new Macro frame)"
        n125 = call <vilib>:"Add State(s) to Queue__jki_lib_state_machine.vi"("State(s) in (\"\")"=w332) -> ("States Out"=w331:string)  [unwired: 14 in]
      }
      frame "Configure: Wait" {
        # "Do not put any code in this frame.\n(It is a separator no-op. You can make a copy of this frame to create a new Macro frame)"
        n126 = call <userlib>:"Wait (ms)__ogtk.vi"("error in (no error)"=w335, "milliseconds to wait"=u32 1000) -> ("error out"=w334:errorcluster)  [unwired: 8 in, 1 out]
        n127 = call <vilib>:"Add State(s) to Queue__jki_lib_state_machine.vi"("State(s) in (\"\")"=w338) -> ("States Out"=w337:string)  [unwired: 14 in]
      }
      frame "---------- Measure ----------" {
        # "Template Separator\n(You can make a copy of, or modify, this frame)"
        n128 = call <vilib>:"Add State(s) to Queue__jki_lib_state_machine.vi"("State(s) in (\"\")"=w342) -> ("States Out"=w341:string)  [unwired: 14 in]
      }
      frame "Measure: Temperature" {
        # "Your code here.\n(You can make a copy of, or modify, this frame)"
        n129 = Unbundle By Name(w350) -> ("Control Experiment"=w345:refnum<class "SMO.Control Experiment.lvclass">, "Instruments.Temperature"=w352:refnum<class "Instrument.Cryostat.lvclass">)
        n130 = call-dynamic "Get Temperature.vi"("error in (no error)"=w351, "Instrument.Cryostat in"=w352) -> ("error out"=w347:errorcluster, "Temperature (K)"=w343:dbl)  [unwired: 5 in, 3 out]
        "T (mK)" <- w343
        n131 = call "Write Dictionary Element.vi"("error in (no error)"=w347, "value"=w343, "key"="Temperature", "Control Experiment in"=w345) -> ("error out"=w346:errorcluster, "Control Experiment out"=w344:refnum<class "Control Experiment.lvclass">)  [unwired: 6 in]
        n132 = Bundle By Name(cluster=w350, "Control Experiment"=w344) -> (w349:T4)
        n133 = call <vilib>:"Add State(s) to Queue__jki_lib_state_machine.vi"("State(s) in (\"\")"=w354) -> ("States Out"=w353:string)  [unwired: 14 in]
      }
      frame "Measure: Magnet" {
        # "Your code here.\n(You can make a copy of, or modify, this frame)"
        n134 = Unbundle By Name(w363) -> ("Control Experiment"=w358:refnum<class "SMO.Control Experiment.lvclass">, "Instruments.Magnet"=w364:refnum<class "Instrument.Cryostat.lvclass">)
        n135 = call-dynamic "Get Magnet Field.vi"("error in (no error)"=w360, "Instrument.Cryostat in"=w364) -> ("error out"=w361:errorcluster, "B Field (T)"=w357:dbl)  [unwired: 5 in, 3 out]
        "Field (T)" <- w357
        n136 = call "Write Dictionary Element.vi"("error in (no error)"=w361, "value"=w357, "key"="Magnet", "Control Experiment in"=w358) -> ("error out"=w355:errorcluster, "Control Experiment out"=w359:refnum<class "Control Experiment.lvclass">)  [unwired: 6 in]
        n137 = Bundle By Name(cluster=w363, "Control Experiment"=w359) -> (w362:T4)
        n138 = call <vilib>:"Add State(s) to Queue__jki_lib_state_machine.vi"("State(s) in (\"\")"=w366) -> ("States Out"=w365:string)  [unwired: 14 in]
      }
      frame "Measure: Capacitance" {
        # "Your code here.\n(You can make a copy of, or modify, this frame)"
        n139 = Unbundle By Name(w367) -> ("Control Experiment"=w373:refnum<class "SMO.Control Experiment.lvclass">, "C Bridge"=w376)
        n140 = call-dynamic "Get Capacitance.vi"("error in (no error)"=w370, "Instrument.CBridge in"=w376) -> ("error out"=w374:errorcluster, "Capacitance (pF)"=w375:dbl)  [unwired: 7 in, 1 out]
        n141 = call "Write Dictionary Element.vi"("error in (no error)"=w374, "value"=w375, "key"="Capacitance", "Control Experiment in"=w373) -> ("error out"=w369:errorcluster, "Control Experiment out"=w371:refnum<class "Control Experiment.lvclass">)  [unwired: 6 in]
        n142 = Bundle By Name(cluster=w367, "Control Experiment"=w371) -> (w372:T4)
        n143 = call <vilib>:"Add State(s) to Queue__jki_lib_state_machine.vi"("State(s) in (\"\")"=w378) -> ("States Out"=w377:string)  [unwired: 14 in]
      }
      frame "Measure: Lockin" {
        n144 = Unbundle By Name(w386) -> ("Control Experiment"=w383:refnum<class "SMO.Control Experiment.lvclass">, "Instruments.Lockin"=w388:refnum<class "Instrument.Lockin.lvclass">)
        n145 = call <userlib>:"waitForNewResults.vi"("error in (no error)"=w389, "Instrument.Lockin in"=w388) -> ("error out"=w382:errorcluster, "Results (Dictionary)"=w379:cluster{"key":string, "value":dbl}[])  [unwired: 7 in, 1 out]
        n146 = call "Results (Dictionary) to X and Y Arrays.vi"("Results (Dictionary)"=w379) -> ("Y"=w384:dbl[], "X"=w385:dbl[])  [unwired: 9 in]
        n147 = for {
          tunnel: w385 -> [w401] mode=indexing
          tunnel: w384 -> [w395] mode=indexing
          tunnel: w382 -> [w394]
          tunnel: [w393] -> w381
          shift-right: [w392] -> w380
          shift-left: w383 -> [w404]
          i -> [w407]
          n148 = Increment(x=w407) -> (x+1=w399:i32)
          n149 = Format Into String(format string="X%d" ("wavenames"), error in=w394, w399) -> (resulting string=w403:string, error out=w398:errorcluster)  [unwired: 1 in]
          n150 = call "Append Dictionary Element.vi"("error in (no error)"=w398, "value"=w401, "key"=w403, "Control Experiment in"=w404) -> ("error out"=w397:errorcluster, "Control Experiment out"=w400:refnum<class "Control Experiment.lvclass">)  [unwired: 6 in]
          n151 = Format Into String(format string="Y%d" ("wavenames"), error in=w397, w399) -> (resulting string=w402:string, error out=w396:errorcluster)  [unwired: 1 in]
          n152 = call "Append Dictionary Element.vi"("error in (no error)"=w396, "value"=w395, "key"=w402, "Control Experiment in"=w400) -> ("error out"=w393:errorcluster, "Control Experiment out"=w392:refnum<class "Control Experiment.lvclass">)  [unwired: 6 in]
        }
        n153 = Bundle By Name(cluster=w386, "Results (Dictionary)"=w379, "Control Experiment"=w380) -> (w387:T4)
        n154 = call <vilib>:"Add State(s) to Queue__jki_lib_state_machine.vi"("State(s) in (\"\")"=w391) -> ("States Out"=w390:string)  [unwired: 14 in]
      }
      frame "Measure: Time" {
        # "Your code here.\n(You can make a copy of, or modify, this frame)"
        n155 = Unbundle By Name(w414) -> ("Control Experiment"=w413:refnum<class "SMO.Control Experiment.lvclass">)
        n156 = Get Date/Time In Seconds() -> (seconds since 1Jan1904=w416:timestamp)
        n157 = To Double Precision Float(number=w416) -> (double precision float=w412:dbl)
        n158 = call "Write Dictionary Element.vi"("error in (no error)"=w410, "value"=w412, "key"="Time", "Control Experiment in"=w413) -> ("error out"=w409:errorcluster, "Control Experiment out"=w408:refnum<class "Control Experiment.lvclass">)  [unwired: 6 in]
        n159 = Bundle By Name(cluster=w414, "Control Experiment"=w408) -> (w415:T4)
        n160 = call <vilib>:"Add State(s) to Queue__jki_lib_state_machine.vi"("State(s) in (\"\")"=w418) -> ("States Out"=w417:string)  [unwired: 14 in]
      }
      frame "---------- File ----------" {
        # "Template Separator\n(You can make a copy of, or modify, this frame)"
        n161 = call <vilib>:"Add State(s) to Queue__jki_lib_state_machine.vi"("State(s) in (\"\")"=w422) -> ("States Out"=w421:string)  [unwired: 14 in]
      }
      frame "File: Configure" {
        # "Template Separator\n(You can make a copy of, or modify, this frame)"
        n162 = call <vilib>:"Add State(s) to Queue__jki_lib_state_machine.vi"("State(s) in (\"\")"=w426) -> ("States Out"=w425:string)  [unwired: 14 in]
      }
      frame "File: Save" {
        # "Template Separator\n(You can make a copy of, or modify, this frame)"
        n163 = Unbundle By Name(w432) -> ("Control Experiment"=w431:refnum<class "SMO.Control Experiment.lvclass">, "Execution:State"=w428:T5)
        n164 = call "Exec State to Append.vi"("Execution:State"=w428) -> ("append?"=w427:bool)  [unwired: 2 in]
        n165 = call "Save Transport TDMS File.vi"("error in (no error)"=w430, 10:w427, "Control Experiment in"=w431) -> ("error out"=w429:errorcluster)  [unwired: 7 in, 1 out]
        n166 = call <vilib>:"Add State(s) to Queue__jki_lib_state_machine.vi"("State(s) in (\"\")"=w434) -> ("States Out"=w433:string)  [unwired: 14 in]
      }
    }
  }
  n167 = call <userlib>:"Tick Count (ms)__ogtk.vi"("error in (no error)"=w5) -> ("error out"=→"error out":errorcluster, "millisecond timer value"=w3:u32)  [unwired: 9 in]
  n168 = Subtract(x=w3, y=w2) -> (x-y=→"x-y":u32)
  n169 = Unbundle By Name(w9) -> ("Transport"=→"Transport out":refnum<class "SMO.Transport.lvclass">)
